vi "Get Parameters.vi"(11 "Process in":refnum<class "Process.lvclass">) -> (2 "Parameters":variant, 3 "Process out":refnum<class "Process.lvclass">)   [LabVIEW 2019, in "TimingDRV Engine.lvlib" / "Process.lvclass"]
uses:
  Process.lvclass
  Process.lvclass/Process.ctl
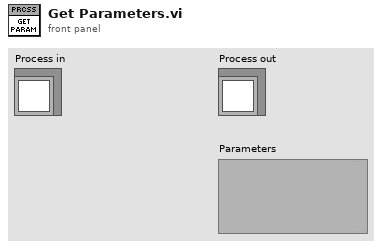
[diagram p1: front panel]
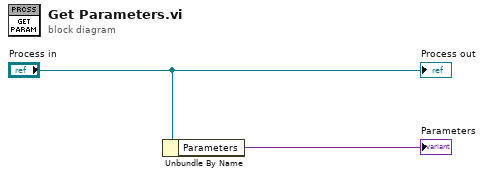
[diagram p0: block diagram]
diagram:
  n1 = Unbundle By Name("Process in") -> ("Parameters"=→"Parameters":variant)
  "Process out" <- "Process in"
